vi "Write error.vi"(0 "error in (no error)":errorcluster) -> ()   [LabVIEW 2015, in "AIT 429 Engine.lvlib"]
uses:
  AIT 429 Engine.lvlib
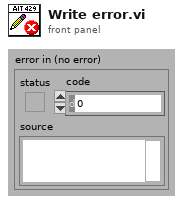
[diagram p1: front panel]
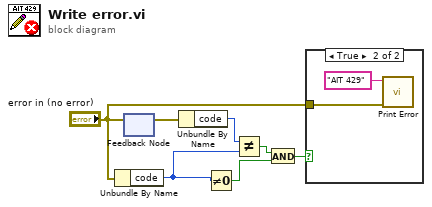
[diagram p0: block diagram]
diagram:
  n1 = Unbundle By Name("error in (no error)") -> ("code"=w2:i32)
  n2 = feedback #1() -> (w4:errorcluster)  [unwired: 1 in]
  n3 = feedback-in #1("error in (no error)") -> ()
  n4 = Unbundle By Name(w4) -> ("code"=w3:i32)
  n5 = Not Equal To 0?(x=w2) -> (x != 0?=w1:bool)
  n6 = Not Equal?(x=w3, y=w2) -> (x != y?=w6:bool)
  n7 = And(x=w6, y=w1) -> (x .and. y?=w5:bool)
  n8 = case shown="True" w5 {
    tunnel: "error in (no error)" -> [_ w9]
    frame False {
    }
    frame True {
      n9 = call "Print Error.vi"("error out"=w9, "Your code's public name"="AIT 429") -> ()  [unwired: 9 in]
    }
  }
